vi "Read Target Destination VI.vi"(8 "error in (no error)":errorcluster, 11 "RIO Target Configuration in":refnum<class "RIO Target Configuration.lvclass">) -> (0 "error out":errorcluster, 2 "Destination VI":path, 3 "RIO Target Configuration out":refnum<class "RIO Target Configuration.lvclass">)   [LabVIEW 2014, in "RIO Target Configuration.lvclass"]
uses:
  RIO Target Configuration.lvclass
  RIO Target Configuration.lvclass/RIO Target Configuration.ctl
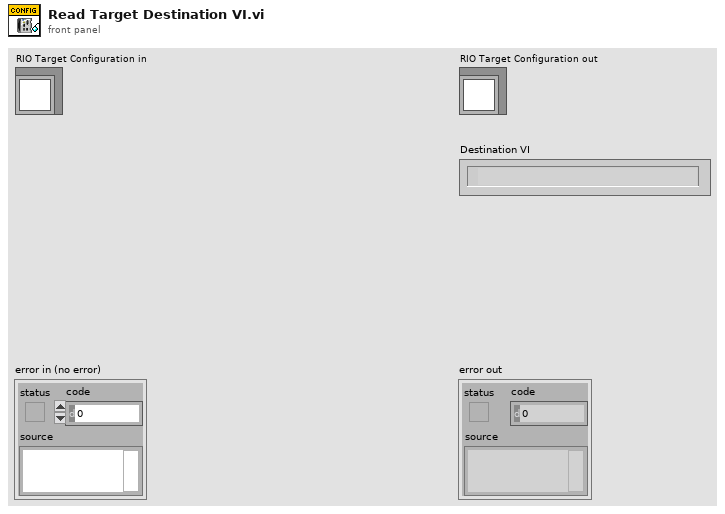
[diagram p1: front panel]
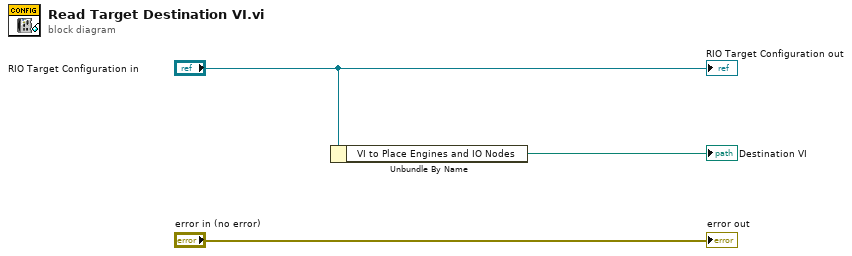
[diagram p0: block diagram]
diagram:
  n1 = Unbundle By Name("RIO Target Configuration in") -> ("VI to Place Engines and IO Nodes"=→"Destination VI":path)
  "error out" <- "error in (no error)"
  "RIO Target Configuration out" <- "RIO Target Configuration in"
